vi "Query Limit Test Results.vi"(8 "error in (no error)":errorcluster, 9 "Limit Test Number":u16=1 min=1 max=2 step=1, 10 "Function":u16(ring) items=["Voltage: DC", "Voltage: AC", "Current: DC", "Current: AC", "2W Resistance", "4W Resistance", "Diode", "Capacitance", "Temperature", "Continuity", "Frequency", "Period", "Ratio", "Digitize Voltage", "Digitize Current"], 11 "VISA resource name":refnum<visa-resource-name>) -> (0 "error out":errorcluster, 1 "Test Results":T1(ring), 2 "Test Passed":bool, 3 "VISA resource name out":refnum<visa-resource-name>)   [LabVIEW 2016, in "Keithley DMM7510.lvlib"]
doc: "This VI queries the results of a limit test.\nThe results:\nTest passed; the measurement is between the upper and lower limits\nTest failed; the measurement exceeded the upper limit\nTest failed; the measurement exceeded the lower limit\nTest failed; the measurement exceeded both limits"
uses:
  Keithley DMM7510.lvlib
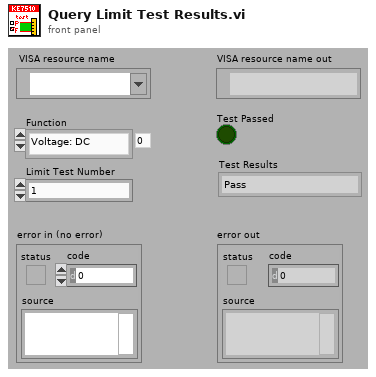
[diagram p1: front panel]
types:
  T1 = enum16{"Pass", "Failed Upper Limit", "Failed Lower Limit", "Failed Both Limits"}
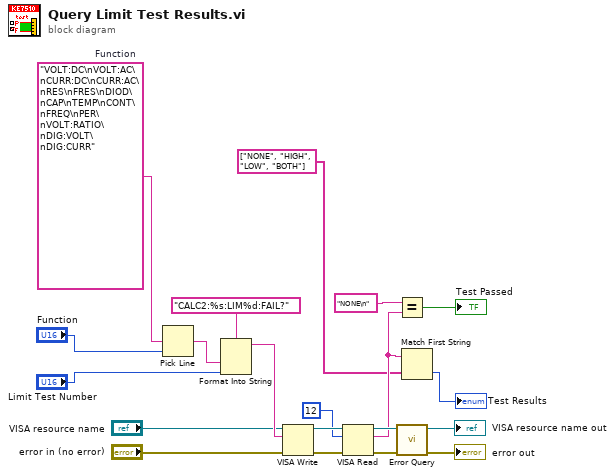
[diagram p0: block diagram]
diagram:
  w6 = "VOLT:DC\nVOLT:AC\nCURR:DC\nCURR:AC\nRES\nFRES\nDIOD\nCAP\nTEMP\nCONT\nFREQ\nPER\nVOLT:RATIO\nDIG:VOLT\nDIG:CURR"  # Function
  n1 = Pick Line(multi-line string=w6, line index="Function") -> (output string=w8:string)  [unwired: 1 out]
  n2 = Format Into String(format string="CALC2:%s:LIM%d:FAIL?", w8, "Limit Test Number") -> (resulting string=w17:string)  [unwired: 2 in, 1 out]
  n3 = VISA Write(VISA resource name="VISA resource name", write buffer=w17, error in (no error)="error in (no error)") -> (VISA resource name out=w13:refnum<visa-resource-name>, error out=w14:errorcluster)  [unwired: 1 out]
  n4 = VISA Read(VISA resource name=w13, byte count=u32 12, error in (no error)=w14) -> (VISA resource name out=w12:refnum<visa-resource-name>, read buffer=w3:string, error out=w11:errorcluster)  [unwired: 1 out]
  n5 = Equal?(x="NONE\n", y=w3) -> (x = y?=→"Test Passed":bool)
  n6 = call "Error Query.vi"("error in (no error)"=w11, "VISA resource name"=w12) -> ("error out"=→"error out":errorcluster, "VISA resource name out"=→"VISA resource name out":refnum<visa-resource-name>)  [unwired: 8 out]
  n7 = Match First String(2:string[] ["NONE", "HIGH", "LOW", "BOTH"], 3:w3) -> (0:→"Test Results":i32)  [unwired: 1 out]
